vi "多通道并行实测.vi"() -> ()   [LabVIEW 2020]
uses:
  <vilib>/Utility/sysdir.llb/System Directory Type.ctl
  <vilib>/Utility/error.llb/DialogType.ctl
  GlobalVariable.vi
  global/SettingVariable.vi
  <vilib>/Analysis/polynomials.llb/Scalar Polynomial Evaluation (DBL).vi
  <vilib>/Analysis/NI_AALPro.lvlib
panel:
  out "T2周期":dbl[](array[numeric]) caption="倍增周期 (s):"
  in  "拟合数":i32(knob)=5 scale=5.0..100.0
  out "多通道并行测量":dbl[][](graph) caption="Waveform Chart - Dark"
  out "四路VO":dbl[](array[numeric]) caption="四路电压输出(V)："
  out "反应性OUT":dbl[](array[numeric])
  out "源与本底开":bool
  in  "源与本底":bool
  out "滤波开":bool
  in  "通量滤波":bool
  out "DRWM开":bool
  in  "动态刻棒":bool
  in  "全量程衔接设置":bool
  in  "添加备注说明":string caption="添加备注说明："
  in  "停止测量":bool
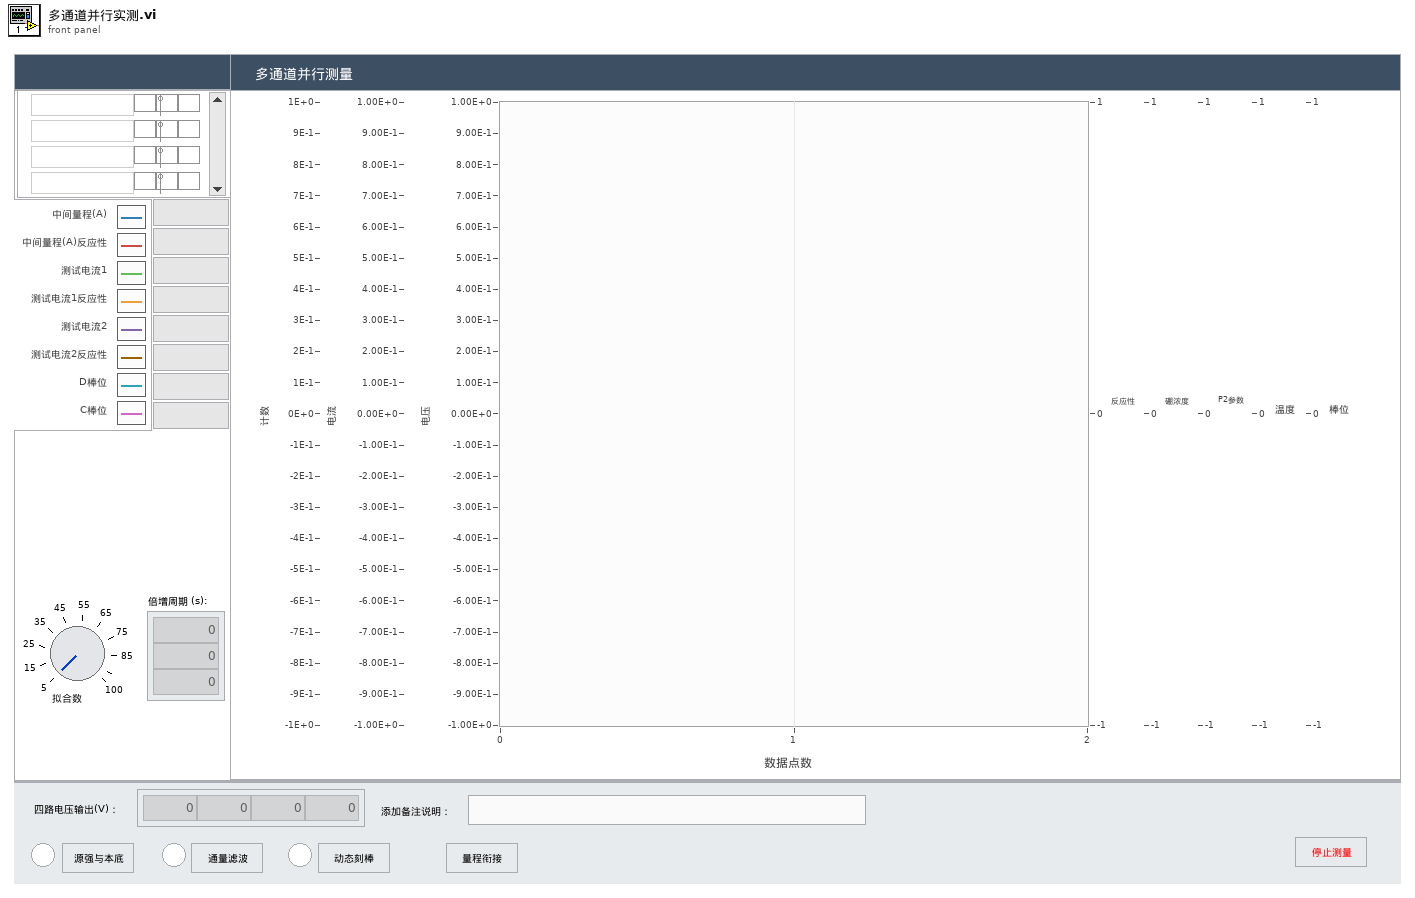
[diagram p1: front panel]
types:
  T1 = enum8{"Enabled", "Disabled", "Disabled and Grayed Out"}
  T2 = enum16{"open", "open or create", "create or replace", "create", "open (read only)"}
  T3 = cluster{"switch":bool, "name":string, "voltage upper":i32, "voltage lower":i32, "physics upper":dbl, "physics lower":dbl, "scale":u16}[]
  T4 = typedef "DialogType.ctl" = u16
  T5 = typedef "System Directory Type.ctl" = i32
  T6 = cluster{"switch":bool, "voltage upper":i32, "voltage lower":i32, "physics upper":dbl, "physics lower":dbl, "input":u16, "log":bool}[]
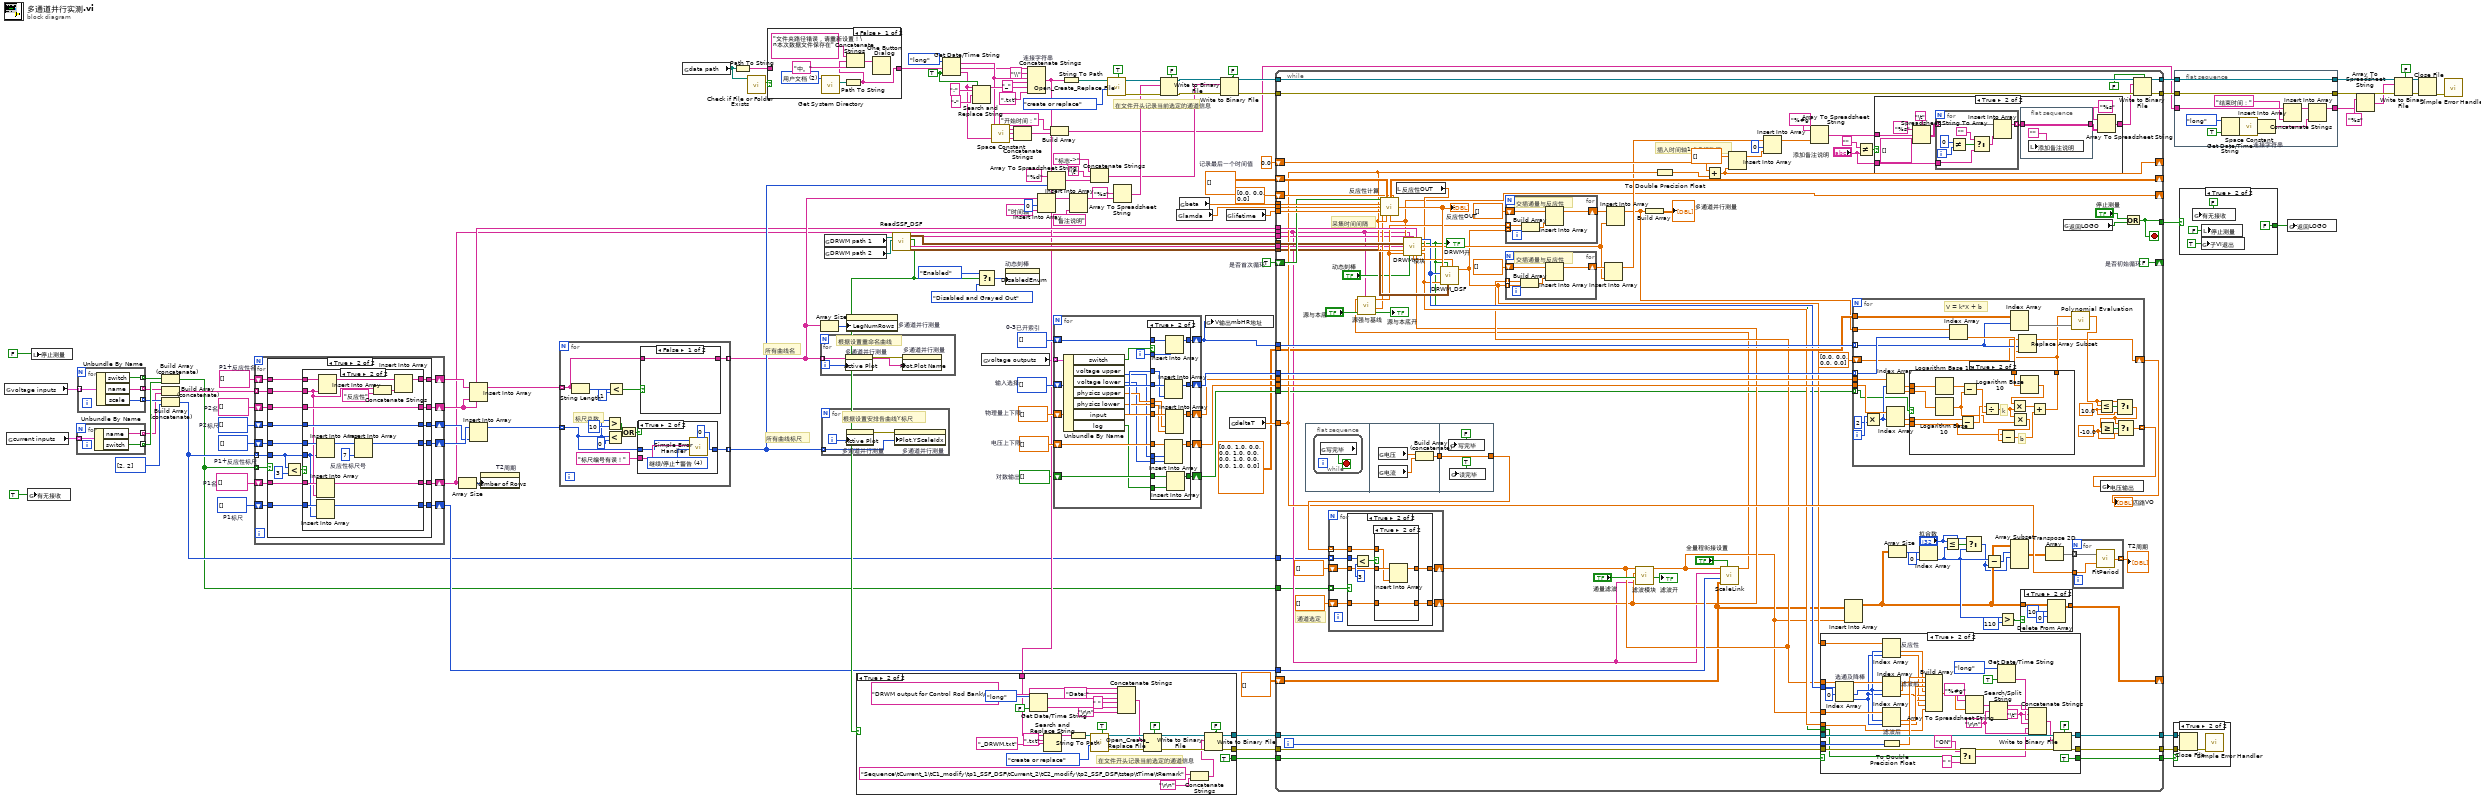
[diagram p0: block diagram]
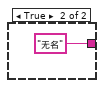
[diagram p3: hidden frame]
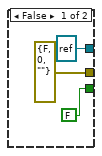
[diagram p5: hidden frame]
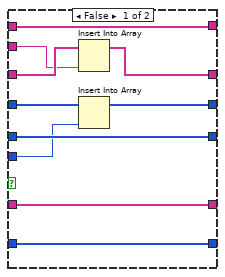
[diagram p9: hidden frame]
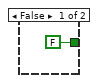
[diagram p10: hidden frame]
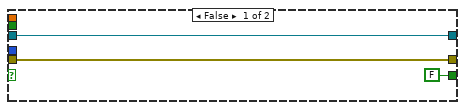
[diagram p11: hidden frame]
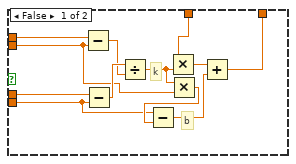
[diagram p13: hidden frame]
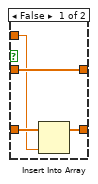
[diagram p16: hidden frame]
diagram:
  w12 = i32[] []  # P1标尺
  w13 = string[] []  # P1名
  w32 = bool[] []  # 对数输出
  w56 = i32[] []  # 0-3已开索引
  w61 = sgl[] []  # 电压上下限
  w62 = sgl[] []  # 物理量上下限
  w63 = u16[] []  # 输入选择
  w79 = TRUE ("需要秒？(F)")
  w84 = 0.0  # 记录最后一个时间值
  w104 = string[] []  # P2名
  w103 = i32[] []  # P2标尺
  w105 = i32[] []  # P1+反应性标尺
  w106 = string[] []  # P1+反应性名
  w108 = TRUE  # 是否首次循环
  # "所有曲线标尺"
  # "所有曲线名"
  # "在文件开头记录当前选定的通道信息"
  n1 = global read "SettingVariable.vi" "voltage inputs"() -> (w22:T3)
  n2 = global read "SettingVariable.vi" "current inputs"() -> (w21:cluster{"name":string, "switch":bool}[])
  n3 = global write "GlobalVariable.vi" "有无接收"(TRUE ("写完毕")) -> ()
  n4 = local write "停止测量"(FALSE ("stop")) -> ()
  n5 = for {
    tunnel: w21 -> [w126] mode=indexing
    tunnel: [w125] -> w16 mode=indexing
    tunnel: [w124] -> w19 mode=indexing
    n6 = Unbundle By Name(w126) -> ("name"=w125:string, "switch"=w124:bool)
  }
  n7 = for {
    tunnel: w22 -> [w130] mode=indexing
    tunnel: [w129] -> w20 mode=indexing
    tunnel: [w128] -> w18 mode=indexing
    tunnel: [w127] -> w17 mode=indexing
    n8 = Unbundle By Name(w130) -> ("switch"=w129:bool, "name"=w128:string, "scale"=w127:u16)
  }
  n9 = Build Array (concatenate)(w20, w19) -> (w8:bool[])
  n10 = Build Array (concatenate)(w18, w16) -> (w14:string[])
  n11 = Build Array (concatenate)(w17, u16[] [2, 2] ("array")) -> (w9:u16[])
  n12 = for {
    tunnel: w14 -> [w137] mode=indexing
    shift-right: [w145] -> w102
    shift-left: w106 -> [w144]
    shift-right: [w142] -> w101
    shift-left: w105 -> [w143]
    shift-right: [w140] -> w54
    shift-left: w104 -> [w141]
    shift-right: [w138] -> w100
    shift-left: w103 -> [w139]
    tunnel: w8 -> [w136] mode=indexing
    tunnel: w9 -> [w135] mode=indexing
    shift-right: [w133] -> w11
    shift-left: w13 -> [w134]
    shift-right: [w131] -> w10
    shift-left: w12 -> [w132]
    n13 = case shown="True" w136 {
      tunnel: [w151 w167] -> w145
      tunnel: w144 -> [w151 w163]
      tunnel: w137 -> [_ w162]
      tunnel: [w150 w165] -> w142
      tunnel: w143 -> [w150 w157]
      tunnel: w141 -> [w149 w161]
      tunnel: [w149 w160] -> w140
      tunnel: w139 -> [w148 w159]
      tunnel: [w148 w158] -> w138
      tunnel: w135 -> [_ w156]
      tunnel: w134 -> [w147 w155]
      tunnel: [w147 w154] -> w133
      tunnel: w132 -> [w146 w153]
      tunnel: [w146 w152] -> w131
      frame False {
      }
      frame True {
        n14 = Less?(x=w156, y=3) -> (x < y?=w164:bool)
        n15 = case shown="True" w164 {
          tunnel: w163 -> [w176 w189]
          tunnel: [w176 w194] -> w167
          tunnel: w157 -> [w177 w185]
          tunnel: [w177 w193] -> w165
          tunnel: w162 -> [w173 w182]
          tunnel: w161 -> [w175 w187]
          tunnel: [w174 w187] -> w160
          tunnel: [w170 w186] -> w158
          tunnel: w159 -> [w172 w186]
          tunnel: w156 -> [w171 w178]
          tunnel: w155 -> [w169 w183]
          tunnel: [w169 w181] -> w154
          tunnel: w153 -> [w168 w180]
          tunnel: [w168 w179] -> w152
          frame False {
            n16 = Insert Into Array(array=w175, new element=w173) -> (w174:string[])  [unwired: 1 in]
            n17 = Insert Into Array(array=w172, new element=w171) -> (w170:i32[])  [unwired: 1 in]
          }
          frame True {
            w190 = 7  # 反应性标尺号
            n18 = Insert Into Array(array=w185, new element=w178) -> (w184:i32[])  [unwired: 1 in]
            n19 = Insert Into Array(array=w183, new element=w182) -> (w181:string[])  [unwired: 1 in]
            n20 = Insert Into Array(array=w180, new element=w178) -> (w179:i32[])  [unwired: 1 in]
            n21 = Insert Into Array(array=w189, new element=w182) -> (w188:string[])  [unwired: 1 in]
            n22 = Insert Into Array(array=w184, new element=w190) -> (w193:i32[])  [unwired: 1 in]
            n23 = Concatenate Strings(w182, "反应性" ("字符串")) -> (w191:string)
            n24 = Insert Into Array(array=w188, new element=w191) -> (w194:string[])  [unwired: 1 in]
          }
        }
      }
    }
  }
  n25 = Array Size(array=w11) -> (size(s)=w50:i32)
  n26 = Insert Into Array(array=w102, new element=w54) -> (w98:string[])  [unwired: 1 in]
  n27 = Insert Into Array(array=w101, new element=w100) -> (w99:i32[])  [unwired: 1 in]
  n28 = property on="T2周期" class="Arr (strict)"("Number of Rows"=w50) -> ()  [unwired: 2 in, 2 out]
  n29 = for {
    tunnel: w99 -> [w200] mode=indexing
    tunnel: w98 -> [w197] mode=indexing
    tunnel: [w198] -> w89 mode=indexing
    tunnel: [w196] -> w55 mode=indexing
    # "标尺总数"
    n30 = String Length(string=w197) -> (length=w202:i32)
    n31 = Greater?(x=w200, y=10) -> (0:w204:bool)
    n32 = Less?(x=w200, y=0) -> (x < y?=w203:bool)
    n33 = Less?(x=w202, y=1) -> (x < y?=w195:bool)
    n34 = Or(x=w204, y=w203) -> (x .or. y?=w201:bool)
    n35 = case shown="True" w201 {
      tunnel: "标尺编号有误！" ("error source (\" \")") -> [_ w212]
      tunnel: w200 -> [w208 w211]
      tunnel: [w208 0] -> w198
      frame False {
      }
      frame True {
        w210 = T4 4 items=["无对话框", "确定信息", "继续或停止信息", "确定信息＋警告", "继续/停止+警告"] ("type of dialog (OK msg:1)")
        n36 = call <vilib>:"Simple Error Handler.vi"("error code (no error:0)"=w211, "error source (\" \")"=w212, "type of dialog (OK msg:1)"=w210) -> ()  [unwired: 2 in, 5 out]
      }
    }
    n37 = case shown="False" w195 {
      tunnel: w197 -> [w213 _]
      tunnel: [w213 "无名"] -> w196
      frame False {
      }
      frame True {
      }
    }
  }
  n38 = global read "SettingVariable.vi" "data path"() -> (w24:path)
  n39 = Path To String(path=w24) -> (string=w25:string)
  n40 = call <vilib>:"Check if File or Folder Exists.vi"("path"=w24) -> ("file or folder exists?"=w49:bool)  [unwired: 8 in, 2 out]
  n41 = case shown="False" w49 {
    tunnel: w25 -> [_ w221]
    tunnel: [w216 w221] -> w48
    frame False {
      w220 = T5 2 items=["用户目录"=0, "用户桌面"=1, "用户文档"=2, "用户应用程序数据"=3, "用户设置"=4, "用户临时目录"=5, "公共文档"=6, "公共应用程序数据"=7, "公共设置"=8, "公共缓存"=13, "系统核心库"=9, "系统安装库"=10, "应用程序文件"=11, "启动盘根目录"=12] ("system directory type")
      n42 = call <vilib>:"Get System Directory.vi"("system directory type"=w220) -> ("system directory"=w218:path)  [unwired: 10 in]
      n43 = Path To String(path=w218) -> (string=w216:string)
      n44 = Concatenate Strings("文件夹路径错误，请重新设置！\n本次数据文件保存在" ("消息"), w216, "中。" ("字符串")) -> (w219:string)
      n45 = One Button Dialog(message=w219) -> ()  [unwired: 1 in, 1 out]
    }
    frame True {
    }
  }
  n46 = for {
    tunnel: w55 -> [w223] mode=indexing
    i -> [w224]
    # "根据设置重命名曲线"
    n47 = property on="多通道并行测量" class="WFChart (strict)"("Active Plot"=w224) -> (error out=w222:errorcluster)  [unwired: 2 in, 1 out]
    n48 = property on="多通道并行测量" class="WFChart (strict)"(error in=w222, "Plot.Plot Name"=w223) -> ()  [unwired: 1 in, 2 out]
  }
  n49 = Array Size(array=w55) -> (size(s)=w29:i32)
  n50 = for {
    tunnel: w89 -> [w225] mode=indexing
    i -> [w227]
    # "根据设置安排各曲线Y标尺"
    n51 = property on="多通道并行测量" class="WFChart (strict)"("Active Plot"=w227) -> (error out=w226:errorcluster)  [unwired: 2 in, 1 out]
    n52 = property on="多通道并行测量" class="WFChart (strict)"(error in=w226, "Plot.YScaleIdx"=w225) -> ()  [unwired: 1 in, 2 out]
  }
  n53 = global read "SettingVariable.vi" "DRWM path 1"() -> (w3:path)
  n54 = global read "SettingVariable.vi" "DRWM path 2"() -> (w2:path)
  n55 = property on="多通道并行测量" class="WFChart (strict)"("LegNumRows"=w29) -> ()  [unwired: 2 in, 2 out]
  n56 = call "ReadSSF_DSF.vi"("DRWM path 2"=w2, "DRWM path 1"=w3) -> ("DSF"=w43:cluster{"x":dbl, "y":dbl}[][], "因子棒号"=w42:string[], "SF_0K"=w33:bool, "SSF"=w44:cluster{"x":dbl, "y":dbl}[][], "文件INFO"=w41:string)  [unwired: 5 in]
  n57 = Get Date/Time String(date format (0)=enum16{"short", "long", "abbreviated"}."long" ("日期格式(0)"), want seconds? (F)=w79) -> (date string=w77:string, time string=w76:string)  [unwired: 1 in]
  n58 = Search and Replace String(replace all?=w79, input string=w76, search string=":", replace string="-" ("replace string (\"\")")) -> (result string=w118:string)  [unwired: 4 in, 3 out]
  n59 = Select(t=T1."Enabled" ("禁用"), s=w33, f=T1."Disabled and Grayed Out" ("禁用")) -> (s? t:f=w47:T1)
  n60 = global read "SettingVariable.vi" "voltage outputs"() -> (w4:T6)
  n61 = call <vilib>:"Space Constant.vi"() -> ("String"=w78:string)
  n62 = property on="动态刻棒" class="Bool"("DisabledEnum"=w47) -> ()  [unwired: 2 in, 2 out]
  n63 = Concatenate Strings ("连接字符串")(w77, w78, w76) -> (w74:string)
  n64 = Concatenate Strings "连接字符串"(w48, "\\" ("字符串"), w77, "_" ("string"), w118, ".txt" ("string")) -> (w36:string)
  n65 = case shown="True" w33 {
    tunnel: [refnum<file> refnum ("refnum out") w241] -> w40
    tunnel: [errorcluster {"status"=FALSE, "code"=0, "source"=""} ("error out") w240] -> w39
    tunnel: w36 -> [_ w239]
    tunnel: [FALSE ("预置数组或字符串大小？(T)") TRUE ("预置数组或字符串大小？(T)")] -> w35
    frame False {
    }
    frame True {
      # "在文件开头记录当前选定的通道信息"
      n66 = Get Date/Time String(date format (0)=enum16{"short", "long", "abbreviated"}."long" ("日期格式(0)"), want seconds? (F)=FALSE ("需要秒？(F)")) -> (date string=w245:string, time string=w243:string)  [unwired: 1 in]
      n67 = Search and Replace String(input string=w239, search string=".txt" ("搜索字符串"), replace string="_DRWM.txt" ("字符串")) -> (result string=w236:string)  [unwired: 5 in, 3 out]
      n68 = String To Path(string=w236) -> (path=w251:path)
      n69 = call <vilib>:"Open_Create_Replace File.vi"("advisory dialog? (display:T)"=TRUE, "function (open:0)"=T2."create or replace", "file path"=w251) -> ("error out"=w258:errorcluster, "refnum"=w256:refnum<file>)  [unwired: 5 in, 2 out]
      n70 = Concatenate Strings("DRWM output for Control Rod Bank\n" ("连接的字符串"), "Date:" ("字符串"), w245, " " ("字符串"), w243, "\r\n") -> (w242:string)
      n71 = Write to Binary File(file (use dialog)=w256, data=w242, error in=w258, 5:FALSE ("预置数组或字符串大小？(T)")) -> (refnum out=w253:refnum<file>, error out=w252:errorcluster)  [unwired: 2 in, 1 out]
      n72 = Concatenate Strings("Sequence\tCurrent_1\tC1_modify\tρ1_SSF_DSF\tCurrent_2\tC2_modify\tρ2_SSF_DSF\tstep\tTime\tRemark" ("连接的字符串"), "\r\n") -> (w233:string)
      n73 = Write to Binary File(file (use dialog)=w253, data=w233, error in=w252, 5:FALSE ("预置数组或字符串大小？(T)")) -> (refnum out=w241:refnum<file>, error out=w240:errorcluster)  [unwired: 2 in, 1 out]
    }
  }
  n74 = Insert Into Array(array=w55, index=0 ("索引"), new element="时间轴" ("新元素/子数组")) -> (w83:string[])
  n75 = Array To Spreadsheet String(array=w89, 3:"%d" ("format string")) -> (spreadsheet string=w88:string)  [unwired: 1 in]
  n76 = Build Array("开始时间：" ("字符串"), w74) -> (w23:string[])
  n77 = for {
    shift-right: [w276] -> w60
    shift-left: w63 -> [w277]
    shift-right: [w272] -> w59
    shift-left: w62 -> [w273]
    shift-right: [w274] -> w58
    shift-left: w61 -> [w275]
    shift-right: [w270] -> w1
    shift-left: w56 -> [w271]
    shift-right: [w267] -> w31
    shift-left: w32 -> [w268]
    tunnel: w4 -> [w266] mode=indexing
    i -> [w269]
    n78 = Unbundle By Name(w266) -> ("switch"=w265:bool, "voltage upper"=w261:i32, "voltage lower"=w260:i32, "physics upper"=w263:dbl, "physics lower"=w262:dbl, "input"=w264:u16, "log"=w259:bool)
    n79 = case shown="True" w265 {
      tunnel: w277 -> [w282 w299]
      tunnel: [w282 w298] -> w276
      tunnel: w264 -> [_ w297]
      tunnel: w275 -> [w280 w296]
      tunnel: [w280 w295] -> w274
      tunnel: w273 -> [w281 w294]
      tunnel: [w281 w293] -> w272
      tunnel: w263 -> [_ w292]
      tunnel: w262 -> [_ w291]
      tunnel: w261 -> [_ w290]
      tunnel: w260 -> [_ w289]
      tunnel: w271 -> [w279 w288]
      tunnel: w269 -> [_ w287]
      tunnel: [w279 w286] -> w270
      tunnel: w259 -> [_ w285]
      tunnel: w268 -> [w278 w284]
      tunnel: [w278 w283] -> w267
      frame False {
      }
      frame True {
        n80 = Insert Into Array(array=w299, new element=w297) -> (w298:u16[])  [unwired: 1 in]
        n81 = Insert Into Array(array=w296, new element #1=w290, new element #2=w289) -> (w295:sgl[])  [unwired: 1 in]
        n82 = Insert Into Array(array=w288, new element=w287) -> (w286:i32[])  [unwired: 1 in]
        n83 = Insert Into Array(array=w294, new element #1=w292, new element #2=w291) -> (w293:sgl[])  [unwired: 1 in]
        n84 = Insert Into Array(array=w284, new element=w285) -> (w283:bool[])  [unwired: 1 in]
      }
    }
  }
  n85 = String To Path(string=w36) -> (path=w51:path)
  n86 = Insert Into Array(array=w83, new element="备注说明" ("新元素/子数组")) -> (w82:string[])  [unwired: 1 in]
  n87 = Concatenate Strings("标志->" ("字符串"), "\t", w88) -> (w85:string)
  n88 = call <vilib>:"Open_Create_Replace File.vi"("advisory dialog? (display:T)"=TRUE, "function (open:0)"=T2."create or replace", "file path"=w51) -> ("error out"=w115:errorcluster, "refnum"=w111:refnum<file>)  [unwired: 5 in, 2 out]
  n89 = Array To Spreadsheet String(array=w82, 3:"%s" ("format string")) -> (spreadsheet string=w107:string)  [unwired: 1 in]
  n90 = Write to Binary File(file (use dialog)=w111, data=w107, error in=w115, 5:FALSE ("预置数组或字符串大小？(T)")) -> (refnum out=w93:refnum<file>, error out=w92:errorcluster)  [unwired: 2 in, 1 out]
  n91 = global read "SettingVariable.vi" "lamda"() -> (w26:dbl[])
  n92 = global read "SettingVariable.vi" "beta"() -> (w27:dbl[])
  n93 = global write "GlobalVariable.vi" "V输出mbHR地址"(w1) -> ()
  n94 = Write to Binary File(file (use dialog)=w93, data=w85, error in=w92, 5:FALSE ("预置数组或字符串大小？(T)")) -> (refnum out=w91:refnum<file>, error out=w90:errorcluster)  [unwired: 2 in, 1 out]
  n95 = global read "SettingVariable.vi" "lifetime"() -> (w28:dbl)
  n96 = global read "SettingVariable.vi" "deltaT"() -> (w6:dbl)
  n97 = while {
    shift-right: [w394] -> _
    shift-left: sgl[][] [] -> [w395]
    tunnel: w27 -> [w396]
    tunnel: w26 -> [w401]
    tunnel: w28 -> [w393]
    shift-right: [w400] -> _
    shift-left: w108 -> [w388]
    tunnel: w91 -> [w392]
    tunnel: w90 -> [w399]
    tunnel: [w357] -> w116
    tunnel: [w398] -> w113
    tunnel: w6 -> [w353]
    tunnel: [w391] -> w109
    shift-right: [w380] -> _
    shift-left: w84 -> [w383]
    shift-right: [w307] -> _
    shift-left: sgl[] [0.0, 0.0, 0.0] ("N(0)OUT") -> [w373]
    shift-right: [w364] -> _
    shift-left: dbl[][] [] ("data") -> [w319]
    tunnel: w60 -> [w368]
    tunnel: w59 -> [w367]
    tunnel: w58 -> [w366]
    tunnel: w1 -> [w365]
    tunnel: w10 -> [w360]
    tunnel: w44 -> [w358]
    tunnel: w43 -> [w351]
    tunnel: w54 -> [w359]
    tunnel: w11 -> [w305]
    tunnel: dbl[][] [[0.0, 1.0, 0.0], [0.0, 1.0, 0.0], [0.0, 1.0, 0.0], [0.0, 1.0, 0.0]] -> [w343]
    tunnel: w42 -> [w340]
    tunnel: w41 -> [w339]
    tunnel: w40 -> [w338]
    tunnel: w39 -> [w337]
    tunnel: [w336] -> w38
    tunnel: [w335] -> w37
    tunnel: w35 -> [w329]
    tunnel: [w328] -> w34
    tunnel: w31 -> [w315]
    tunnel: w9 -> [w303]
    tunnel: w8 -> [w304]
    i -> [w332]
    stop <- w357 stop-if-true
    w400 = FALSE  # 是否初始循环
    # "通道选定"
    # "插入时间轴1或多行数据"
    # "采集时间间隔"
    n98 = flat-sequence {
      tunnel: [w403] -> w323
      tunnel: [w407] -> w385
      tunnel: w323 -> [w407]
      frame #0 {
        n99 = while {
          stop <- w402 stop-if-true
          n100 = global read "GlobalVariable.vi" "写完毕"() -> (w402:bool)
        }
      }
      frame #1 {
        n101 = global read "GlobalVariable.vi" "电压"() -> (w405:dbl[])
        n102 = global read "GlobalVariable.vi" "电流"() -> (w404:dbl[])
        n103 = Build Array (concatenate)(w405, w404) -> (w403:dbl[])
      }
      frame #2 {
        n104 = global write "GlobalVariable.vi" "写完毕"(FALSE ("写完毕")) -> ()
        n105 = global write "GlobalVariable.vi" "读完毕"(TRUE ("写完毕")) -> ()
      }
    }
    n106 = for {
      shift-right: [w540] -> w322
      shift-left: dbl[] [] ("data") -> [w541]
      shift-right: [w538] -> w321
      shift-left: dbl[] [] ("data") -> [w539]
      tunnel: w385 -> [w537] mode=indexing
      tunnel: w304 -> [w536] mode=indexing
      tunnel: w303 -> [w535] mode=indexing
      n107 = case shown="True" w536 {
        tunnel: w535 -> [_ w550]
        tunnel: w541 -> [w543 w548]
        tunnel: [w543 w547] -> w540
        tunnel: w539 -> [w542 w546]
        tunnel: [w542 w545] -> w538
        tunnel: w537 -> [_ w544]
        frame False {
        }
        frame True {
          n108 = Less?(x=w550, y=3) -> (x < y?=w549:bool)
          n109 = case shown="True" w549 {
            tunnel: w548 -> [w553 w558]
            tunnel: [w553 w557] -> w547
            tunnel: w546 -> [w555 w559]
            tunnel: [w554 w559] -> w545
            tunnel: w544 -> [w552 w556]
            frame False {
              n110 = Insert Into Array(array=w555, new element=w552) -> (w554:dbl[])  [unwired: 1 in]
            }
            frame True {
              n111 = Insert Into Array(array=w558, new element=w556) -> (w557:dbl[])  [unwired: 1 in]
            }
          }
        }
      }
    }
    n112 = local read "反应性OUT"() -> (w326:dbl[])
    n113 = call "滤波模块.vi"("通量名称"=w305, "执行:调用时显示前面板"="通量滤波", "P2信号"=w321, "通量in"=w322) -> ("滤波开"=→"滤波开":bool, "通量out"=w320:dbl[])  [unwired: 5 in, 1 out]
    n114 = To Double Precision Float(number=w353) -> (double precision float=w316:dbl)
    n115 = Add(x=w383, y=w316) -> (x+y=w380:dbl)
    n116 = call "ScaleLink.vi"("执行:调用时显示前面板"="全量程衔接设置", "曲线输入"=w319, "通量标尺"=w360, "通量名称"=w305, "通量输入"=w320) -> ("通量输出"=w300:dbl[])  [unwired: 6 in]
    n117 = call "源强与基线.vi"("通量名称"=w305, "执行:调用时显示前面板"="源与本底", "通量in"=w300) -> ("源与基线灯"=→"源与本底开":bool, "源强out"=w341:dbl[], "通量out"=w346:dbl[])  [unwired: 4 in]
    n118 = call "DRWM模块.vi"("通量名称"=w305, "因子说明"=w339, "P2名称"=w359, "SSF因子"=w358, "因子棒名"=w340, "时间步长"=w353, "反应性in"=w326, "通量in"=w346, "执行:调用时显示前面板"="动态刻棒", "P2信号"=w321) -> ("通量out"=w307:dbl[], "上下段通量索引"=w334:u16[], "DRWM开"=w324:bool, "P2信号out"=w345:dbl[], "棒限"=w342:dbl[], "动态棒位"=w327:dbl)
    "DRWM开" <- w324
    n119 = call "反应性计算.vi"("循环次数"=w388, "λi*Ci(0)"=w395, "N(0)IN"=w373, "βi"=w396, "λi"=w401, "中子寿命"=w393, "源强"=w341, "采集间隔"=w353, "中子注量率"=w307) -> ("λi*Ci(t)"=w394:sgl[][], "反应性OUT"=w352:dbl[])  [unwired: 5 in]
    "反应性OUT" <- w352
    n120 = call "DRWM_DSF.vi"("棒限值"=w342, "DSF因子"=w351, "DRWM开"=w324, "动态棒位"=w327, "上下段通量选择"=w334, "反应性in"=w352) -> ("反应性out"=w333:dbl[])  [unwired: 5 in]
    n121 = for {
      tunnel: w322 -> [w450] mode=indexing
      tunnel: w333 -> [w449] mode=indexing
      shift-right: [w451] -> w347
      shift-left: dbl[] [] ("平滑掉数据") -> [w452]
      # "交插通量与反应性"
      n122 = Build Array(w450, w449) -> (w448:dbl[])
      n123 = Insert Into Array(array=w452, new element=w448) -> (w451:dbl[])  [unwired: 1 in]
    }
    n124 = for {
      tunnel: w346 -> [w562] mode=indexing
      tunnel: w333 -> [w561] mode=indexing
      shift-right: [w563] -> w384
      shift-left: dbl[] [] ("平滑掉数据") -> [w564]
      # "交插通量与反应性"
      n125 = Build Array(w562, w561) -> (w560:dbl[])
      n126 = Insert Into Array(array=w564, new element=w560) -> (w563:dbl[])  [unwired: 1 in]
    }
    n127 = Insert Into Array(array=w347, new element=w345) -> (w344:dbl[])  [unwired: 1 in]
    n128 = Insert Into Array ("数组插入")(array=w384, new element=w345) -> (w317:dbl[])  [unwired: 1 in]
    n129 = Build Array(w317) -> (→"多通道并行测量":dbl[][])
    n130 = Insert Into Array(array=dbl[] [], new element=w380) -> (w381:dbl[])  [unwired: 1 in]
    n131 = Insert Into Array(array=w344, index=0 ("索引 (行)"), new element=w381) -> (w318:dbl[])
    n132 = Array To Spreadsheet String(array=w318, 3:"%#g" ("format string")) -> (spreadsheet string=w375:string)  [unwired: 1 in]
    n133 = case shown="True" w329 {
      tunnel: w338 -> [w411 w446]
      tunnel: w337 -> [w410 w445]
      tunnel: [w411 w444] -> w336
      tunnel: [w410 w443] -> w335
      tunnel: w334 -> [_ w441]
      tunnel: w322 -> [_ w439]
      tunnel: w320 -> [_ w438]
      tunnel: w333 -> [_ w437]
      tunnel: w332 -> [_ w434]
      tunnel: [FALSE ("预置数组或字符串大小？(T)") TRUE ("预置数组或字符串大小？(T)")] -> w328
      tunnel: w327 -> [_ w412]
      tunnel: w324 -> [_ w418]
      frame False {
      }
      frame True {
        w417 = "\r\n"
        w416 = "\t"
        n134 = Index Array "选通及降棒"(array=w441, index #1=0 ("索引")) -> (element #1=w436:u16, element #2=w435:u16)  [unwired: 1 in]
        n135 = Index Array "反应性"(array=w437, index #1=w436, index #2=w435) -> (element #1=w430:dbl, element #2=w427:dbl)
        n136 = Index Array "滤波前"(array=w439, index #1=w436, index #2=w435) -> (element #1=w432:dbl, element #2=w429:dbl)
        n137 = Index Array "滤波后"(array=w438, index #1=w436, index #2=w435) -> (element #1=w431:dbl, element #2=w428:dbl)
        n138 = To Double Precision Float(number=w434) -> (double precision float=w433:dbl)
        n139 = Build Array(w433, w432, w431, w430, w429, w428, w427, w412) -> (w426:dbl[])
        n140 = Select(t="ON" ("format string"), s=w418, f=" " ("format string")) -> (s? t:f=w415:string)
        n141 = Array To Spreadsheet String(array=w426, 3:"%#g" ("format string")) -> (spreadsheet string=w424:string)  [unwired: 1 in]
        n142 = Search/Split String(string=w424, search string/char (-)=w417) -> (substring before match=w425:string)  [unwired: 1 in, 2 out]
        n143 = Get Date/Time String(date format (0)=enum16{"short", "long", "abbreviated"}."long" ("日期格式(0)"), want seconds? (F)=TRUE ("需要秒？(F)")) -> (time string=w420:string)  [unwired: 1 in, 1 out]
        n144 = Concatenate Strings(w425, w416, w420, w416, w415, w417) -> (w423:string)
        n145 = Write to Binary File(file (use dialog)=w446, data=w423, error in=w445, 5:FALSE ("预置数组或字符串大小？(T)")) -> (refnum out=w444:refnum<file>, error out=w443:errorcluster)  [unwired: 2 in, 1 out]
      }
    }
    n146 = Insert Into Array(array=w319, new element=w320) -> (w330:dbl[][])  [unwired: 2 in]
    n147 = for {
      tunnel: w368 -> [w477] mode=indexing
      tunnel: w367 -> [w483]
      tunnel: w366 -> [w482]
      tunnel: w317 -> [w478]
      tunnel: w365 -> [w461] mode=indexing
      tunnel: w343 -> [w467]
      tunnel: w315 -> [w462] mode=indexing
      tunnel: [w463] -> w314 mode=indexing
      shift-right: [w458] -> w301
      shift-left: dbl[] [0.0, 0.0, 0.0, 0.0] ("四路VO") -> [w460]
      i -> [w481]
      w469 = sgl -10.0 ("y")
      w471 = sgl 10.0 ("y")
      # "V = k*X + b"
      n148 = Multiply(x=w481, y=2) -> (x*y=w479:i32)
      n149 = Index Array(array=w483, index #1=w479) -> (element #1=w476:sgl, element #2=w473:sgl)  [unwired: 1 in]
      n150 = Index Array(array=w482, index #1=w479) -> (element #1=w474:sgl, element #2=w465:sgl)  [unwired: 1 in]
      n151 = Index Array(array=w478, index=w477) -> (element=w475:dbl)
      n152 = case shown="True" w462 {
        tunnel: w476 -> [w495 w504]
        tunnel: w475 -> [w492 w498]
        tunnel: w474 -> [w491 w500]
        tunnel: w473 -> [w489 w503]
        tunnel: w465 -> [w485 w499]
        tunnel: [w484 w496] -> w459
        frame False {
          # "b"
          # "k"
          n153 = Subtract(x=w495, y=w489) -> (x-y=w493:sgl)
          n154 = Subtract(x=w491, y=w485) -> (x-y=w494:sgl)
          n155 = Divide(x=w494, y=w493) -> (x/y=w490:sgl)
          n156 = Multiply(x=w492, y=w490) -> (x*y=w487:dbl)
          n157 = Multiply(x=w490, y=w489) -> (x*y=w488:sgl)
          n158 = Subtract(x=w485, y=w488) -> (x-y=w486:sgl)
          n159 = Add(x=w487, y=w486) -> (x+y=w484:dbl)
        }
        frame True {
          # "b"
          # "k"
          n160 = Logarithm Base 10(1:w504) -> (0:w502:sgl)
          n161 = Logarithm Base 10(1:w503) -> (0:w501:sgl)
          n162 = Subtract(x=w500, y=w499) -> (x-y=w505:sgl)
          n163 = Subtract(x=w502, y=w501) -> (x-y=w506:sgl)
          n164 = Divide(x=w505, y=w506) -> (x/y=w507:sgl)
          n165 = Multiply(x=w507, y=w501) -> (x*y=w508:sgl)
          n166 = Subtract(x=w499, y=w508) -> (x-y=w510:sgl)
          n167 = Logarithm Base 10(1:w498) -> (0:w497:dbl)
          n168 = Multiply(x=w497, y=w507) -> (x*y=w509:dbl)
          n169 = Add(x=w509, y=w510) -> (x+y=w496:dbl)
        }
      }
      n170 = Index Array(array=w467, index (row)=w461) -> (element=w466:dbl[])  [unwired: 1 in]
      n171 = Replace Array Subset(array=w460, new element=w459, index=w461) -> (w458:dbl[])
      n172 = call-poly <vilib>:"Polynomial Evaluation.vi"("P(x)"=w466, "a"=w459) -> ("P(a)"=w464:dbl)  [unwired: 1 out]
      n173 = Less Or Equal?(x=w464, y=w471) -> (x <= y?=w472:bool)
      n174 = Select(t=w464, s=w472, f=w471) -> (s? t:f=w468:dbl)
      n175 = Greater Or Equal?(x=w468, y=w469) -> (x >= y?=w470:bool)
      n176 = Select(t=w468, s=w470, f=w469) -> (s? t:f=w463:dbl)
    }
    "四路VO" <- w301
    n177 = Not Equal?(x="", y="添加备注说明") -> (x != y?=w376:bool)
    n178 = case shown="True" w376 {
      tunnel: [w514 w515] -> w374
      tunnel: "添加备注说明" -> [_ w524]
      tunnel: w375 -> [w514 w519]
      frame False {
      }
      frame True {
        n179 = Spreadsheet String To Array(delimiter (Tab)="\t", format string="%s", spreadsheet string=w519, array type (2D Dbl)=string[][] [] ("添加的数组")) -> (array=w520:string[][])
        n180 = for {
          tunnel: w520 -> [w534] mode=indexing
          tunnel: [w533] -> w518 mode=indexing
          tunnel: w524 -> [w528]
          i -> [w532]
          n181 = Not Equal?(x=0 ("y"), y=w532) -> (x != y?=w530:bool)
          n182 = Select(t="", s=w530, f=w528) -> (s? t:f=w529:string)
          n183 = Insert Into Array(array=w534, new element=w529) -> (w533:string[])  [unwired: 1 in]
        }
        n184 = flat-sequence {
          tunnel: w518 -> [w525]
          tunnel: [w525] -> w516
          frame #0 {
            n185 = local write "添加备注说明"("") -> ()
          }
        }
        n186 = Array To Spreadsheet String(array=w516, 3:"%s" ("format string")) -> (spreadsheet string=w515:string)  [unwired: 1 in]
      }
    }
    n187 = Array Size(array=w330) -> (size(s)=w372:i32[])
    n188 = Index Array(array=w372, index=0 ("索引")) -> (element=w331:i32)
    n189 = Less Or Equal?(x="拟合数", y=w331) -> (x <= y?=w370:bool)
    n190 = Select(t="拟合数", s=w370, f=w331) -> (s? t:f=w312:i32)
    n191 = Subtract(x=w331, y=w312) -> (x-y=w313:i32)
    n192 = Greater?(x=w331, y=110) -> (0:w362:bool)
    n193 = Array Subset ("数组子集")(array=w330, index (row)=w313, length (row)=w312) -> (w310:dbl[][])  [unwired: 2 in]
    n194 = case shown="True" w362 {
      tunnel: w330 -> [w453 w457]
      tunnel: [w453 w456] -> w364
      frame False {
      }
      frame True {
        n195 = Delete From Array ("删除数组元素")(array=w457, length=10 ("y"), index (row)=0 ("索引 (行)")) -> (array with subset deleted=w456:dbl[][])  [unwired: 1 in, 1 out]
      }
    }
    n196 = Transpose 2D Array(2D array=w310) -> (transposed array=w311:dbl[][])
    n197 = global read "GlobalVariable.vi" "返回LOGO"() -> (w356:bool)
    n198 = for {
      tunnel: w311 -> [w513] mode=indexing
      tunnel: [w511] -> w308 mode=indexing
      tunnel: w353 -> [w512]
      n199 = call "FitPeriod.vi"("delta"=w512, "curve"=w513) -> ("T2"=w511:dbl)
    }
    "T2周期" <- w308
    n200 = global write "GlobalVariable.vi" "电压输出"(w314) -> ()
    n201 = Or(x="停止测量", y=w356) -> (x .or. y?=w357:bool)
    n202 = Write to Binary File(file (use dialog)=w392, data=w374, error in=w399, 5:FALSE ("预置数组或字符串大小？(T)")) -> (refnum out=w391:refnum<file>, error out=w398:errorcluster)  [unwired: 2 in, 1 out]
  }
  n203 = case shown="True" w34 {
    tunnel: w38 -> [_ w566]
    tunnel: w37 -> [_ w565]
    frame False {
    }
    frame True {
      n204 = Close File(refnum=w566, error in=w565) -> (error out=w567:errorcluster)  [unwired: 1 out]
      n205 = call <vilib>:"Simple Error Handler.vi"("error in (no error)"=w567) -> ()  [unwired: 4 in, 5 out]
    }
  }
  n206 = flat-sequence {
    tunnel: w113 -> [w573]
    tunnel: w109 -> [w574]
    tunnel: w23 -> [w572]
    tunnel: [w574] -> w68
    tunnel: [w573] -> w67
    tunnel: [w568] -> w71
    frame #0 {
      n207 = Get Date/Time String(date format (0)=enum16{"short", "long", "abbreviated"}."long" ("日期格式(0)"), want seconds? (F)=TRUE ("需要秒？(F)")) -> (date string=w577:string, time string=w576:string)  [unwired: 1 in]
      n208 = call <vilib>:"Space Constant.vi"() -> ("String"=w575:string)
      n209 = Concatenate Strings "连接字符串"(w577, w575, w576) -> (w569:string)
      n210 = Insert Into Array(array=w572, new element="结束时间：" ("字符串")) -> (w570:string[])  [unwired: 1 in]
      n211 = Insert Into Array(array=w570, new element=w569) -> (w568:string[])  [unwired: 1 in]
    }
  }
  n212 = case shown="True" w116 {
    tunnel: [FALSE ("返回LOGO") FALSE ("返回LOGO")] -> w53
    frame False {
    }
    frame True {
      n213 = global write "GlobalVariable.vi" "有无接收"(FALSE ("写完毕")) -> ()
      n214 = global write "GlobalVariable.vi" "子VI退出"(TRUE ("子VI退出")) -> ()
      n215 = local write "停止测量"(FALSE ("Exit")) -> ()
    }
  }
  n216 = global write "GlobalVariable.vi" "返回LOGO"(w53) -> ()
  n217 = Array To Spreadsheet String(array=w71, 3:"%s" ("format string")) -> (spreadsheet string=w66:string)  [unwired: 1 in]
  n218 = Write to Binary File(file (use dialog)=w68, data=w66, error in=w67, 5:FALSE ("预置数组或字符串大小？(T)")) -> (refnum out=w70:refnum<file>, error out=w69:errorcluster)  [unwired: 2 in, 1 out]
  n219 = Close File(refnum=w70, error in=w69) -> (error out=w75:errorcluster)  [unwired: 1 out]
  n220 = call <vilib>:"Simple Error Handler.vi"("error in (no error)"=w75) -> ()  [unwired: 4 in, 5 out]
